vi "Read Temperature Setpoint.vi"(8 "error in (no error)":errorcluster, 11 "ThermotronDriver in":refnum<class "ThermotronDriver.lvclass">) -> (0 "error out":errorcluster, 2 "Temperature Setpoint":dbl, 3 "ThermotronDriver out":refnum<class "ThermotronDriver.lvclass">)   [LabVIEW 2023, in "ThermotronDriver.lvlib" / "ThermotronDriver.lvclass"]
uses:
  ThermotronDriver.lvclass
  ThermotronDriver.lvclass/ThermotronDriver.ctl
  <vilib>/ADAS Replay HIL/Channels/Tag Wrapper/Tag Wrapper.lvlib
  <vilib>/ADAS Replay HIL/Channels/Tag Wrapper/Polymorphic/Read Channel (Double).vi
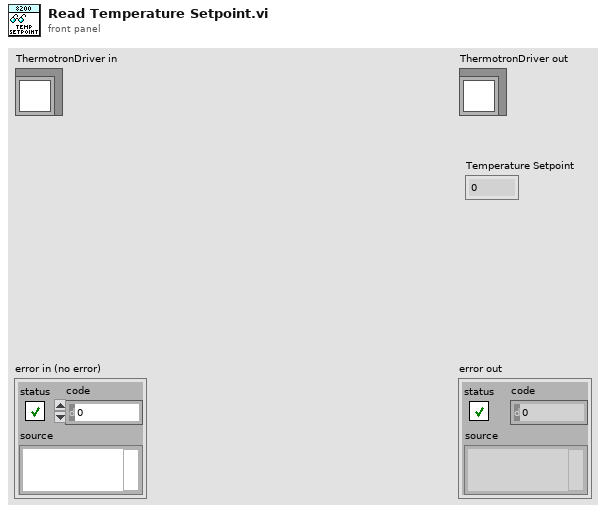
[diagram p1: front panel]
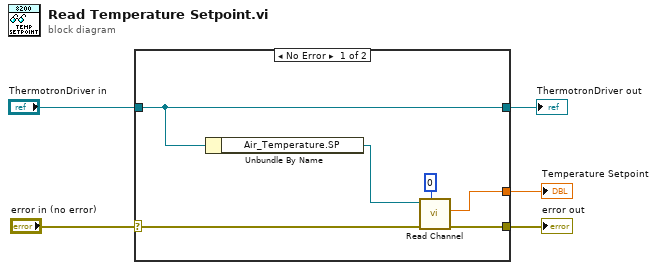
[diagram p0: block diagram]
diagram:
  n1 = case shown="No Error" "error in (no error)" {
    selector: "error in (no error)" -> [w11 w13]
    tunnel: [w10 w13] -> w4
    tunnel: [w8 w12] -> w2
    tunnel: "ThermotronDriver in" -> [w8 w12]
    tunnel: [w9 _] -> w1
    frame No Error {
      n2 = Unbundle By Name(w8) -> ("Air_Temperature.SP"=w7:refnum<k21>)
      n3 = call-poly <vilib>:"Read Channel.vi"("Timeout (ms)"=0, "error in"=w11, "ADAS HIL Channel in"=w7) -> ("error out"=w10:errorcluster, "Value out"=w9:dbl)  [unwired: 5 in, 2 out]
    }
    frame Error {
    }
  }
  "error out" <- w4
  "ThermotronDriver out" <- w2
  "Temperature Setpoint" <- w1
